vi "FMInfoFGV.vi"(1 "GetSetEnum":T3=enum."Get", 2 "FMInfoIn":T1={"buffer size"=0, "bits"=0, "CarrierInfo"={"frequency"=10.0, "amplitude"=1.0, "sample rate"=0, "waveform type"=enum."Sine"}, "ModulatorInfo"={"frequency"=10.0, "amplitude"=1.0, "sample rate"=0, "waveform type"=enum."Sine"}, "Feedback"=FALSE} {"ModulatorInfo"."amplitude" format="%0.2p"; "ModulatorInfo"."frequency" format="%0.2p"; "CarrierInfo"."amplitude" format="%0.2p"; "CarrierInfo"."frequency" format="%0.2p"}) -> (0 "FMInfoOut":T1={"buffer size"=0, "bits"=0, "CarrierInfo"={"frequency"=10.0, "amplitude"=1.0, "sample rate"=0, "waveform type"=enum."Sine"}, "ModulatorInfo"={"frequency"=10.0, "amplitude"=1.0, "sample rate"=0, "waveform type"=enum."Sine"}, "Feedback"=FALSE} {"ModulatorInfo"."amplitude" format="%0.2p"; "ModulatorInfo"."frequency" format="%0.2p"; "CarrierInfo"."amplitude" format="%0.2p"; "CarrierInfo"."frequency" format="%0.2p"})   [LabVIEW 2016]
uses:
  FGV/GetSetEnum.ctl
  Generation/GenerateWaveform/FMInfo.ctl
  Generation/Oscillator/WaveformType.ctl
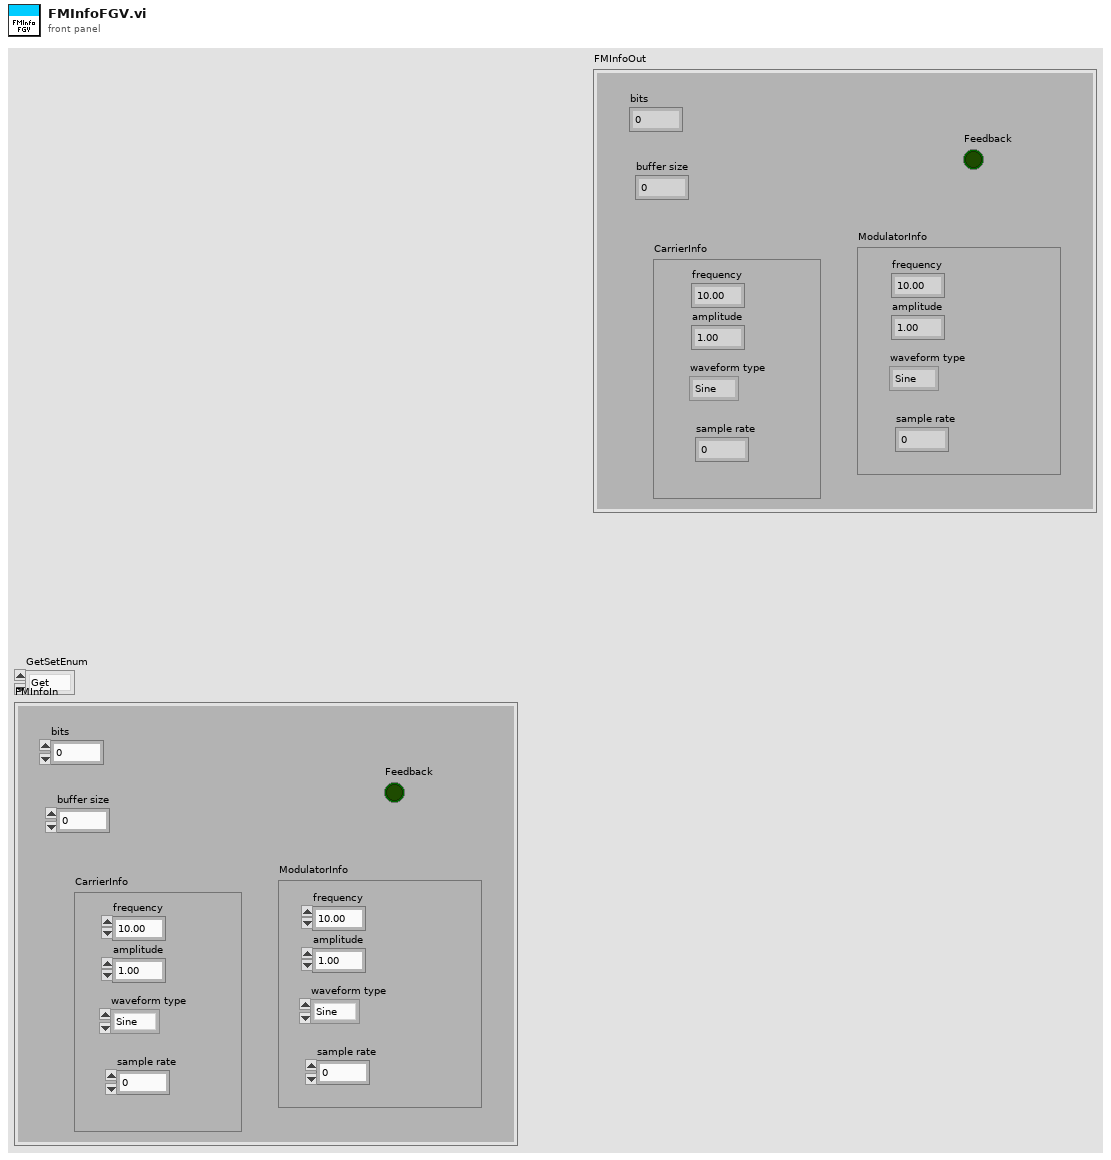
[diagram p1: front panel]
types:
  T1 = typedef "FMInfo.ctl" = cluster{"buffer size":i32, "bits":i32, "CarrierInfo":cluster{"frequency":dbl, "amplitude":dbl, "sample rate":i32, "waveform type":T2}, "ModulatorInfo":cluster{"frequency":dbl, "amplitude":dbl, "sample rate":i32, "waveform type":T2}, "Feedback":bool}
  T2 = typedef "WaveformType.ctl" = enum16{"Sine", "Triangle", "Square", "Sawtooth"}
  T3 = typedef "GetSetEnum.ctl" = enum16{"Init", "Get", "Set"}
  T4 = typedef "ASIOData.ctl" = cluster{"Buffer Config":cluster{"# buffers":i32, "Buffer size":i32, "unit (ms)":enum16{"time (ms)", "Samples"}}, "Format (44kHz, 16Bit, stereo)":cluster{"Rate":i32, "Bits":i32, "Channels":u32}, "Play":bool, "Exit":bool}
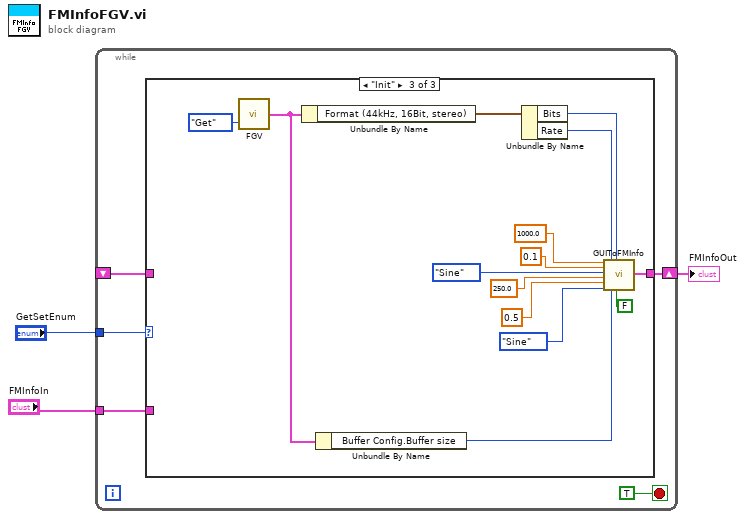
[diagram p0: block diagram]
diagram:
  n1 = while {
    tunnel: "GetSetEnum" -> [w7]
    shift-right: [w5] -> w1
    shift-left: _ -> [w6]
    tunnel: "FMInfoIn" -> [w4]
    stop <- TRUE stop-if-true
    n2 = case shown="\"Init\"" w7 {
      tunnel: w6 -> [w9 _ _]
      tunnel: [w9 w10 w24] -> w5
      tunnel: w4 -> [_ w10 _]
      frame "Get", Default {
      }
      frame "Set" {
      }
      frame "Init" {
        n3 = call "FGV.vi"("GetSetEnum"=GetSetEnum."Get") -> ("ASIODataOut"=w14:T4)  [unwired: 1 in]
        n4 = Unbundle By Name(w14) -> ("Format (44kHz, 16Bit, stereo)"=w22:cluster{"Rate":i32, "Bits":i32, "Channels":u32})
        n5 = Unbundle By Name(w14) -> ("Buffer Config.Buffer size"=w13:i32)
        n6 = Unbundle By Name(w22) -> ("Bits"=w21:i32, "Rate"=w20:i32)
        n7 = call "GUIToFMInfo.vi"("carrier frequency"=1000.0, "amplitude"=0.1, "carrier waveform"=WaveformType."Sine" ("carrier waveform 2"), "modulation frequency"=250.0, "modulation index"=0.5 ("modulation depth"), "modulator waveform"=WaveformType."Sine" ("carrier waveform 2"), "sample rate"=w20, "buffer size"=w13, "bits"=w21, "Feedback"=FALSE) -> ("FMInfo"=w24:T1)  [unwired: 9 in]
      }
    }
  }
  "FMInfoOut" <- w1
